vi "Read Measurement(Single Point).vi"(0 "VISA resource name":refnum<visa-resource-name>, 11 "error in (no error)":errorcluster) -> (4 "VISA resource name out":refnum<visa-resource-name>, 6 "Measurement":dbl, 15 "error out":errorcluster)   [LabVIEW 2020, in "3458A Virtual Digitizer.lvlib" / "3458A Basic Driver.lvlib"]
doc: "Reads and returns a single measurement from the instrument. Note that the instrument starts taking measurements after setting the trigger count except in cases of using an external or level trigger in which case it waits for the adequate input signal."
uses:
  3458A Basic Driver.lvlib
  Low Level/Fetch Measurement(Single Point).vi
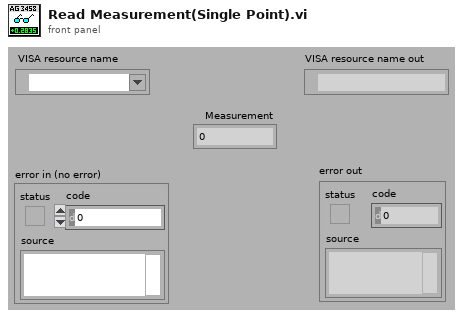
[diagram p1: front panel]
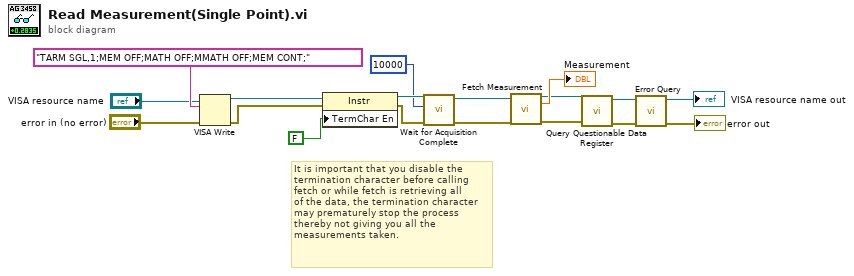
[diagram p0: block diagram]
diagram:
  # "It is important that you disable the \ntermination character before calling\nfetch or while fetch is retrieving all\nof the data, the termination character\nmay prematurely stop the process\nthereby not giving you all the \nmeasurements taken."
  n1 = VISA Write(VISA resource name="VISA resource name", write buffer="TARM SGL,1;MEM OFF;MATH OFF;MMATH OFF;MEM CONT;" ("format string"), error in (no error)="error in (no error)") -> (VISA resource name out=w4:refnum<visa-resource-name>, error out=w3:errorcluster)  [unwired: 1 out]
  n2 = property class="Instr"(reference=w4, error in=w3, "TermChar En"=FALSE) -> (reference out=w13:refnum<visa-resource-name>, error out=w12:errorcluster)
  n3 = call "Wait for Acquisition Complete.vi"("error in (no error)"=w12, "Maximum Time (10000 ms)"=u32 10000, "VISA resource name"=w13) -> ("error out"=w10:errorcluster, "VISA resource name out"=w11:refnum<visa-resource-name>)  [unwired: 7 in]
  n4 = call-poly "Fetch Measurement.vi"("VISA resource name"=w11, "error in (no error)"=w10) -> ("VISA resource name out"=w8:refnum<visa-resource-name>, "Measurement"=→"Measurement":sgl, "error out"=w7:errorcluster)  [unwired: 11 in]
  n5 = call "Query Questionable Data Register.vi"("error in (no error)"=w7, "VISA resource name"=w8) -> ("error out"=w5:errorcluster, "VISA resource name out"=w6:refnum<visa-resource-name>)  [unwired: 7 in, 1 out]
  n6 = call "Error Query.vi"("error in (no error)"=w5, "VISA resource name"=w6) -> ("error out"=→"error out":errorcluster, "VISA resource name out"=→"VISA resource name out":refnum<visa-resource-name>)  [unwired: 6 in, 2 out]
